vi "SL TAGS Get Value By Name.vi"(4 "Tag Scope":T1=enum."Server", 6 "Tag Type":T2, 8 "error in (no error)":errorcluster, 10 "Tag Name":string, 11 "EEISysLink in":refnum<class "EEISysLink.lvclass">) -> (0 "error out":errorcluster, 1 "Found?":bool, 2 "Tag Value":T3, 3 "EEISysLink out":refnum<class "EEISysLink.lvclass">)   [LabVIEW 2017, in "EEISysLink.lvclass"]
doc: "Will return the current value of the first tag that matches the input name. \n\nJames Tillett P.E.\nEndeavor Engineering Inc.\nwww.endeavoreng.com"
uses:
  EEISysLink.lvclass
  Controls/SL Tag Value.ctl
  Controls/SL Tag Data Type.ctl
  Controls/SL Tag Type.ctl
  Controls/SL Tag Scope.ctl
  EEISysLink.lvclass/EEISysLink.ctl
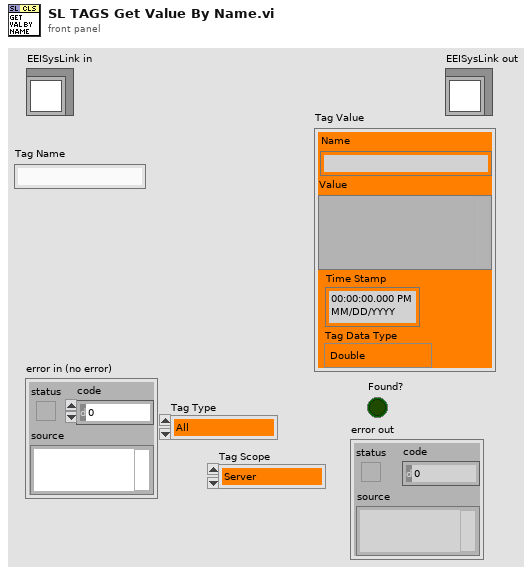
[diagram p1: front panel]
types:
  T1 = typedef "EEISysLink.lvclass/SL Tag Scope.ctl" = enum16{"Local", "Server"}
  T2 = typedef "EEISysLink.lvclass/SL Tag Type.ctl" = enum16{"All", "Supervisor", "Worker"}
  T3 = typedef "SL Tag Value.ctl" = cluster{"Value":variant, "Time Stamp":timestamp, "Tag Data Type":T4, "Name":string}
  T4 = typedef "EEISysLink.lvclass/SL Tag Data Type.ctl" = enum16{"Double", "Integer", "String", "Boolean", "Waveform"}
  T5 = typedef "EEISysLink.lvclass/SL Tag.ctl" = cluster{"Class Properties":T6, "SL Tag":refnum<class "NI Skyline Tag.lvclass">, "SystemLink Cluster":T9, "Class Value":variant}
  T6 = typedef "EEISysLink.lvclass/SL Tag Properties.ctl" = cluster{"Class Data Type":T4, "Name":string, "Description":string, "Interpolation Method":T7, "Unit of Measure":T8, "Maximum Interpolation":string, "Role":T2}
  T7 = typedef "EEISysLink.lvclass/SL Tag Interpolation Method.ctl" = enum16{"linear", "pilinear", "step"}
  T8 = typedef "EEISysLink.lvclass/SL Tag Unit of Measure.ctl" = enum16{"no units", "Second", "Hour", "Minute", "Day", "Year", "Month", "Week", "Foot", "Yard", "Meter", "Centimeter", "Inch", "Mile", "Nautical Mile", "Miles per Hour", "Meters per second", "Square meter", "Cubic meter", "Cubic centimeter", "Cubic inch", "Liter", "Gallon", "Gallons dry US", "Gallon UK", "Percent", "Revolutions per minute", "Revolution", "Degree angle", "Astronomical Unit", "Atom", "Atomic mass", "Bar", "Byte", "C (speed of light)", "Curie", "Decibel", "Electron Volt", "Ounce", "Knot", "G", "Grade", "Are", "Hectare", "Faraday", "Franklin", "Gilbert", "Erg", "Lambert", "Maxwell", "Gauss", "Electron mass", "Kilogram force", "Pound force", "Rad", "Centiradian", "Sphere", "Mach", "Fluid Ounces", "Fluid Ounces UK", "Fahrenheit", "Celsius", "Kelvin", "Rankine", "Gram", "Kilogram", "Pound", "Short/US Ton", "Long/UK ton", "Metric ton", "Mole", "Pounds per square inch", "Inches water column", "Torr", "Millitorr", "Millimeter mercury", "Inches mercury", "Bar (2)", "Atmosphere", "Pascal", "Watt", "kiloWatt", "Horsepower", "Kilowatt Hour", "British thermal units", "Millions of BTU", "Ampere", "Candela", "Radian", "Steradian", "Bit", "Hertz", "Newton", "Joule", "Coulomb", "Volt", "Farad", "Ohm", "Siemens", "Weber", "Tesla", "Henry", "Lumen", "Lux", "Becqueral", "Gray", "Sievert", "Katal", "Angstrom", "Light Year", "Parsec", "Point", "Pixel", "Dyne", "Kilogram force (2)", "Pound force (2)", "Rem", "Rutherford", "Roentgen"}
  T9 = typedef "NI Skyline Tag.lvlib/Tag Cluster.ctl" = cluster{"Path":string, "Data Type":T10, "Value":variant, "Time Stamp":timestamp}
  T10 = typedef "NI Skyline Tag.lvlib/DataType.ctl" = enum32{"Double", "Integer", "String"}
  T11 = typedef "NI Skyline Tag.lvlib/Aggregates Double.ctl" = cluster{"Count":i32, "Max":dbl, "Min":dbl, "Mean":dbl}
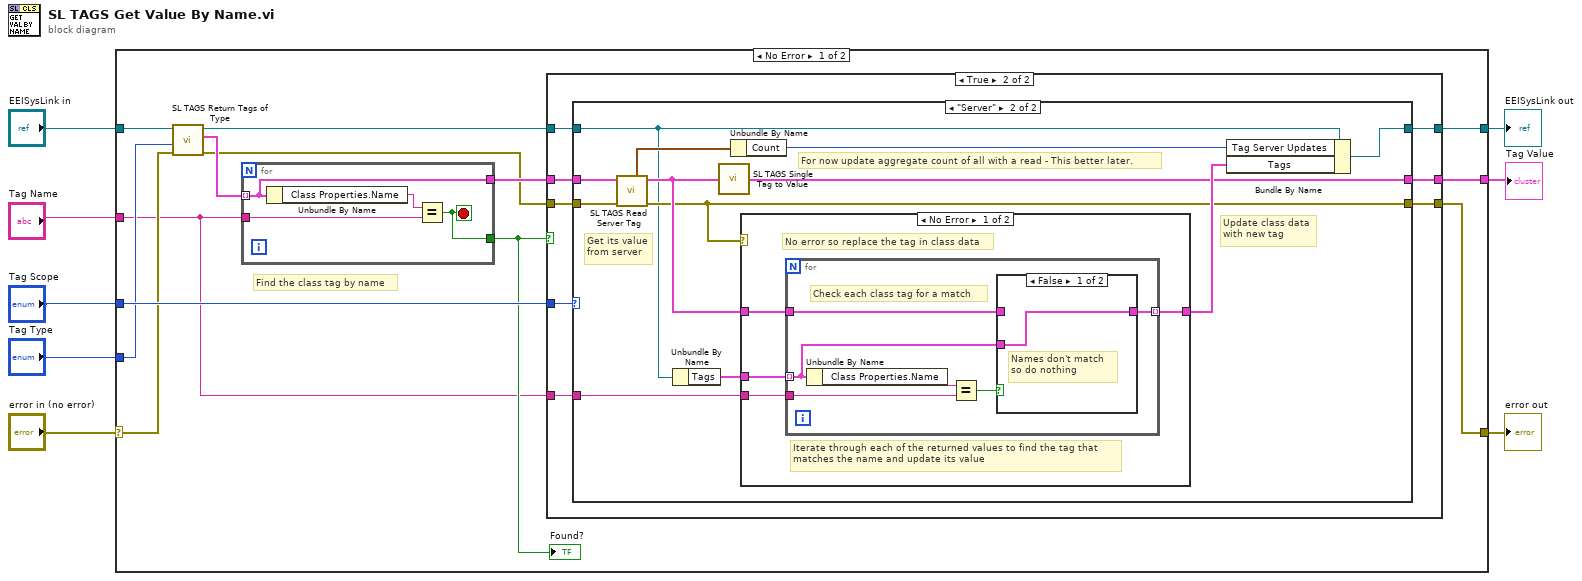
[diagram p0: block diagram]
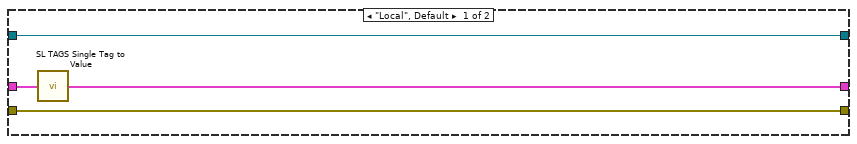
[diagram p3: hidden frame]
diagram:
  n1 = case shown="No Error" "error in (no error)" {
    selector: "error in (no error)" -> [w16 w66]
    tunnel: [w10 w66] -> w7
    tunnel: [w20 w65] -> w5
    tunnel: "EEISysLink in" -> [w19 w65]
    tunnel: "Tag Scope" -> [w21 _]
    tunnel: "Tag Type" -> [w15 _]
    tunnel: "Tag Name" -> [w12 _]
    tunnel: [w9 _] -> w1
    frame No Error {
      # "Find the class tag by name"
      n2 = call "SL TAGS Return Tags of Type.vi"("error in (no error)"=w16, "Tag Type"=w15, "EEISysLink in"=w19) -> ("error out"=w11:errorcluster, "Tags of Type"=w17:T5[], "EEISysLink out"=w18:refnum<class "EEISysLink.lvclass">)  [unwired: 6 in]
      n3 = for {
        tunnel: w17 -> [w62] mode=indexing
        tunnel: w12 -> [w64]
        tunnel: [w62] -> w13
        tunnel: [w61] -> w14
        stop <- w61 stop-if-true
        n4 = Unbundle By Name(w62) -> ("Class Properties.Name"=w63:string)
        n5 = Equal?(x=w63, y=w64) -> (x = y?=w61:bool)
      }
      "Found?" <- w14
      n6 = case shown="True" w14 {
        tunnel: w21 -> [_ w31]
        tunnel: [w23 w30] -> w20
        tunnel: w18 -> [w23 w29]
        tunnel: w13 -> [_ w28]
        tunnel: w12 -> [_ w27]
        tunnel: [_ w26] -> w9
        tunnel: w11 -> [w22 w25]
        tunnel: [w22 w24] -> w10
        frame False {
          # "Tag not found"
        }
        frame True {
          n7 = case shown="\"Server\"" w31 {
            tunnel: w29 -> [w35 w37]
            tunnel: [w35 w46] -> w30
            tunnel: w28 -> [w34 w44]
            tunnel: w27 -> [_ w43]
            tunnel: [w33 w41] -> w26
            tunnel: w25 -> [w32 w40]
            tunnel: [w32 w39] -> w24
            frame "Local", Default {
              n8 = call "SL TAGS Single Tag to Value.vi"("Tag"=w34) -> ("Tag Value"=w33:T3)  [unwired: 4 in]
            }
            frame "Server" {
              # "For now update aggregate count of all with a read - This better later."
              # "Get its value\nfrom server"
              # "Update class data\nwith new tag"
              n9 = call "SL TAGS Read Server Tag.vi"("error in (no error)"=w40, "Tag Ref In"=w44) -> ("error out"=w39:errorcluster, "Tag Ref Out"=w42:T5, "Aggregate Values"=w38:T11)  [unwired: 7 in]
              n10 = Unbundle By Name(w37) -> ("Tags"=w47:T5[])
              n11 = call "SL TAGS Single Tag to Value.vi"("Tag"=w42) -> ("Tag Value"=w41:T3)  [unwired: 4 in]
              n12 = Unbundle By Name(w38) -> ("Count"=w36:i32)
              n13 = case shown="No Error" w39 {
                tunnel: w47 -> [w51 w60]
                tunnel: [w50 w60] -> w45
                tunnel: w43 -> [w49 _]
                tunnel: w42 -> [w48 _]
                frame No Error {
                  # "Iterate through each of the returned values to find the tag that\nmatches the name and update its value"
                  # "No error so replace the tag in class data"
                  n14 = for {
                    tunnel: w51 -> [w54] mode=indexing
                    tunnel: w48 -> [w55]
                    tunnel: [w53] -> w50 mode=indexing
                    tunnel: w49 -> [w52]
                    # "Check each class tag for a match"
                    n15 = Unbundle By Name(w54) -> ("Class Properties.Name"=w57:string)
                    n16 = Equal?(x=w57, y=w52) -> (x = y?=w56:bool)
                    n17 = case shown="False" w56 {
                      tunnel: w55 -> [_ w59]
                      tunnel: w54 -> [w58 _]
                      tunnel: [w58 w59] -> w53
                      frame False {
                        # "Names don't match\nso do nothing"
                      }
                      frame True {
                        # "Match so replace\nwith updated tag"
                      }
                    }
                  }
                }
                frame Error {
                  # "Error on update so don't change tag values"
                }
              }
              n18 = Bundle By Name(cluster=w37, "Tag Server Updates"=w36, "Tags"=w45) -> (w46:refnum<class "EEISysLink.lvclass">)
            }
          }
        }
      }
    }
    frame Error {
    }
  }
  "error out" <- w7
  "EEISysLink out" <- w5
  "Tag Value" <- w1
